vi "CheckFileName.vi"(8 "error in":errorcluster, 10 "Path String":string, 11 "Path":path) -> (0 "error out":errorcluster, 1 "Offset to Bad Character(s)":i32[](array[numeric]), 2 "Bad Character(s)":string, 3 "Bad Filename?":bool, 5 "Path String Out":string)   [LabVIEW 2020]
doc: "This vi will check a file name for invalid characters. Either a path or a string can be input. If both are input the path will take precedence. If neither is input this vi will generate an error. Any bad characters found are output in a srting and can be added to a message to notify a user what characters in their file name are bad.\nR.Fogg NTS Corp 505-345-9499"
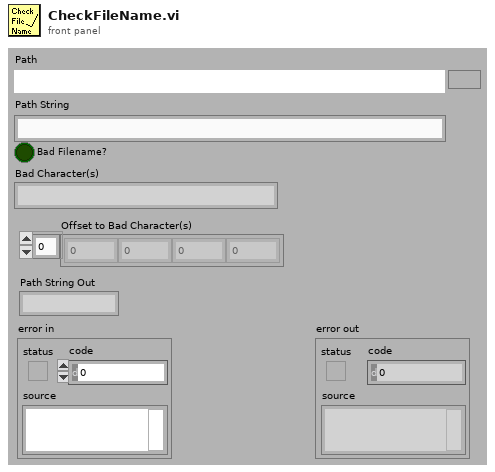
[diagram p1: front panel]
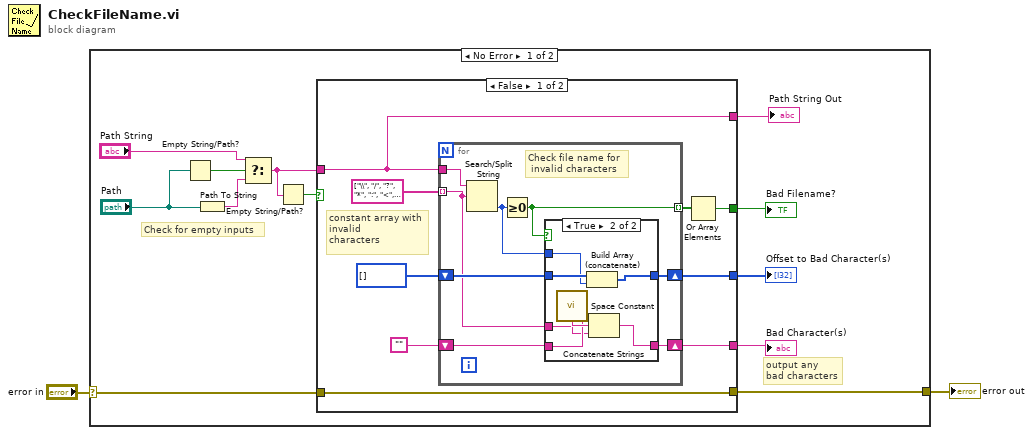
[diagram p0: block diagram]
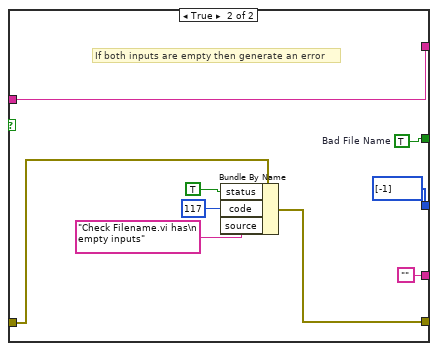
[diagram p3: hidden frame]
diagram:
  n1 = case shown="No Error" "error in" {
    selector: "error in" -> [w7 w50]
    tunnel: [w6 w50] -> w1
    frame No Error {
      # "output any \nbad characters"
      # "Check for empty inputs"
      n2 = Empty String/Path?(string/path="Path") -> (empty?=w14:bool)
      n3 = Path To String(path="Path") -> (string=w12:string)
      n4 = Select(t="Path String", s=w14, f=w12) -> (s? t:f=w9:string)
      n5 = Empty String/Path?(string/path=w9) -> (empty?=w10:bool)
      n6 = case shown="False" w10 {
        tunnel: w9 -> [w16 w41]
        tunnel: [w21 ""] -> w8
        tunnel: [w20 w49] -> w5
        tunnel: w7 -> [w19 w47]
        tunnel: [w19 w43] -> w6
        tunnel: [w18 i32[] [-1]] -> w4
        tunnel: [w16 w41] -> w3
        frame False {
          # "constant array with invalid\ncharacters"
          n7 = for {
            tunnel: w16 -> [w31]
            tunnel: [w30] -> w23 mode=indexing
            shift-right: [w28] -> w21
            shift-left: "" -> [w29]
            shift-right: [w25] -> w18
            shift-left: i32[] [] -> [w26]
            tunnel: string[] ["\\", "/", "?", "*", ":", "<", ">", "\"", "|"] -> [w24] mode=indexing
            # "Check file name for\n invalid characters"
            n8 = Search/Split String(string=w31, search string/char (-)=w24) -> (offset of match=w27:i32)  [unwired: 1 in, 2 out]
            n9 = Greater Or Equal To 0?(x=w27) -> (x >= 0?=w30:bool)
            n10 = case shown="True" w30 {
              tunnel: w29 -> [w33 w39]
              tunnel: [w33 w37] -> w28
              tunnel: w24 -> [_ w38]
              tunnel: w27 -> [_ w35]
              tunnel: [w32 w34] -> w25
              tunnel: w26 -> [w32 w36]
              frame False {
              }
              frame True {
                n11 = call <vilib>:"Space Constant.vi"() -> ("String"=w40:string)
                n12 = Build Array (concatenate)(w36, w35) -> (w34:i32[])
                n13 = Concatenate Strings(w39, w40, w38) -> (w37:string)
              }
            }
          }
          n14 = Or Array Elements(Boolean array=w23) -> (logical OR=w20:bool)
        }
        frame True {
          w49 = TRUE  # Bad File Name
          # "If both inputs are empty then generate an error"
          n15 = Bundle By Name(cluster=w47, "status"=TRUE, "code"=117, "source"="Check Filename.vi has\n empty inputs") -> (w43:errorcluster)
        }
      }
      "Bad Character(s)" <- w8
      "Bad Filename?" <- w5
      "Offset to Bad Character(s)" <- w4
      "Path String Out" <- w3
    }
    frame Error {
      # "Skip check if error is input"
    }
  }
  "error out" <- w1
